vi "Value Change.vi"(7 "objects":T1, 8 "error in":errorcluster, 11 "Multi Column Listbox in":refnum<class "Multi Column Listbox.lvclass">) -> (0 "error out":errorcluster, 2 "Update?":bool, 3 "Multi Column Listbox out":refnum<class "Multi Column Listbox.lvclass">)   [LabVIEW 2013, in "Table Manager.lvlib" / "Multi Column Listbox.lvclass"]
uses:
  Multi Column Listbox.lvclass
  Table Manager/object ref.ctl
  Configuration Editor/Classes/Engine Parent/Engine Parent Editor Node.lvclass
  Configuration Editor/Classes/Module editor node/module editor node.lvclass
  Table Manager/Table Manager.lvclass/Table Manager.ctl
  Multi Column Listbox.lvclass/Multi Column Listbox.ctl
  Line/Line.lvclass/Line.ctl
  Column/Column.lvclass
  Column/Column.lvclass/Column.ctl
  Table Manager/Read Line.vi
  Read Listbox.vi
  Table Manager/Read Index.vi
  Line/Read Columns.vi
  Table Manager/Table Manager.lvclass
  Line/Line.lvclass
  Table Manager.lvlib
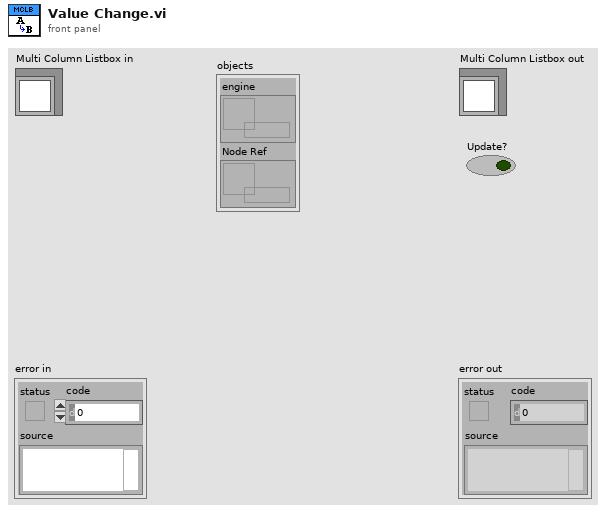
[diagram p1: front panel]
types:
  T1 = typedef "Table Manager.lvlib/Table Manager.lvclass/object ref.ctl" = cluster{"engine":refnum<data-value>, "Node Ref":refnum<data-value>}
  T2 = typedef "Table Manager.lvlib/Cell Change.ctl" = cluster{"row":i32, "col":i32, "old value":string, "new value":string}
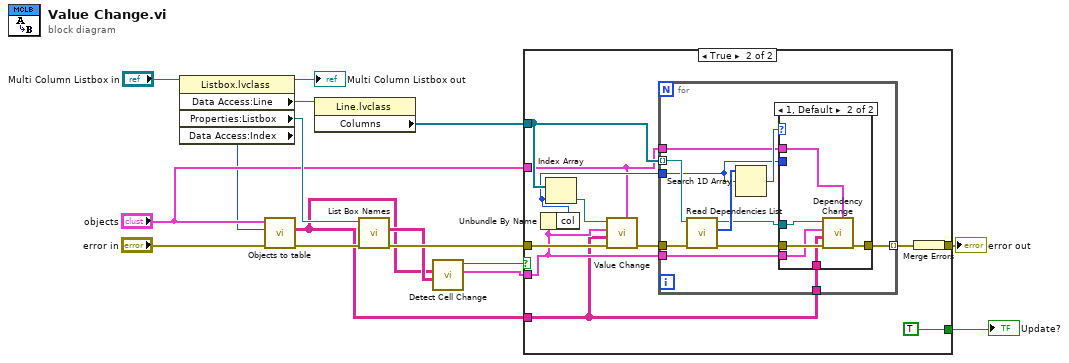
[diagram p0: block diagram]
diagram:
  n1 = property class="Listbox.lvclass"(reference="Multi Column Listbox in") -> (reference out=→"Multi Column Listbox out":refnum<class "Multi Column Listbox.lvclass">, "Data Access:Line"=w11:refnum<class "Line.lvclass">, "Properties:Listbox"=w13:refnum<vi>, "Data Access:Index"=w1:i32)  [unwired: 1 in, 1 out]
  n2 = call "Objects to table.vi"("error in (no error)"="error in", "Table Index"=w1, "object ref in"="objects") -> ("error out"=w16:errorcluster, "table"=w4:string[][])  [unwired: 6 in, 1 out]
  n3 = property class="Line.lvclass"(reference=w11) -> ("Columns"=w9:refnum<class "Column.lvclass">[])  [unwired: 1 in, 2 out]
  n4 = call "List Box Names.vi"("error in (no error)"=w16, "MulticolumnListbox in"=w13) -> ("error out"=w8:errorcluster, "ItemNames"=w6:string[][])  [unwired: 7 in, 1 out]
  n5 = call "Detect Cell Change.vi"("new values"=w6, "old values"=w4) -> ("Cluster"=w3:T2, "value change"=w5:bool)  [unwired: 6 in, 2 out]
  n6 = case shown="True" w5 {
    tunnel: [w17 w26] -> w10
    tunnel: w9 -> [_ w24]
    tunnel: w8 -> [w17 w23]
    tunnel: "objects" -> [_ w21]
    tunnel: w4 -> [_ w19]
    tunnel: w3 -> [_ w20]
    tunnel: [_ TRUE ("Update?")] -> w2
    frame False {
    }
    frame True {
      n7 = Unbundle By Name(w20) -> ("col"=w22:i32)
      n8 = Index Array(array=w24, index=w22) -> (element=w28:refnum<class "Column.lvclass">)
      n9 = call-dynamic "Value Change.vi"("object ref in"=w21, "error in (no error)"=w23, "old values"=w19, "Table Change"=w20, "Column in"=w28) -> ("error out"=w27:errorcluster)  [unwired: 5 in, 1 out]
      n10 = for {
        tunnel: w22 -> [w31]
        tunnel: w27 -> [w35]
        tunnel: [w39] -> w25 mode=indexing
        tunnel: w24 -> [w37] mode=indexing
        tunnel: w21 -> [w32]
        tunnel: w19 -> [w30]
        tunnel: w20 -> [w29]
        n11 = call "Read Dependencies List.vi"("error in (no error)"=w35, "Column in"=w37) -> ("error out"=w34:errorcluster, "Dependecies"=w38:i32[], "Column out"=w36:refnum<class "Column.lvclass">)  [unwired: 7 in]
        n12 = Search 1D Array(1D array=w38, element=w31) -> (index of element=w33:i32)  [unwired: 1 in]
        n13 = case shown="1, Default" w33 {
          tunnel: [w40 w46] -> w39
          tunnel: w34 -> [w40 w45]
          tunnel: w36 -> [_ w44]
          tunnel: w32 -> [_ w43]
          tunnel: w31 -> [_ _]
          tunnel: w30 -> [_ w42]
          tunnel: w29 -> [_ w41]
          frame -1 {
          }
          frame 1, Default {
            n14 = call-dynamic "Dependency Change.vi"("object ref in"=w43, "error in (no error)"=w45, "old values"=w42, "Table Change"=w41, "Column in"=w44) -> ("error out"=w46:errorcluster)  [unwired: 5 in, 1 out]
          }
        }
      }
      n15 = Merge Errors(w25) -> (w26:errorcluster)
    }
  }
  "error out" <- w10
  "Update?" <- w2
